vi "YAML to Elements.vi"(8 "error in (no error)":errorcluster, 10 "Parser State":T4) -> (0 "error out":errorcluster, 2 "Elements":T1[](array[typedef]))   [LabVIEW 2020, in "CDM-Config.lvlib" / "Config-YAML.lvclass"]
uses:
  Config-YAML.lvclass
  Config-YAML.lvclass/Config-YAML.ctl
  Value Type.ctl
  CDM-Config.lvlib
  Parser State.ctl
  Meta Data.ctl
  Config Element.ctl
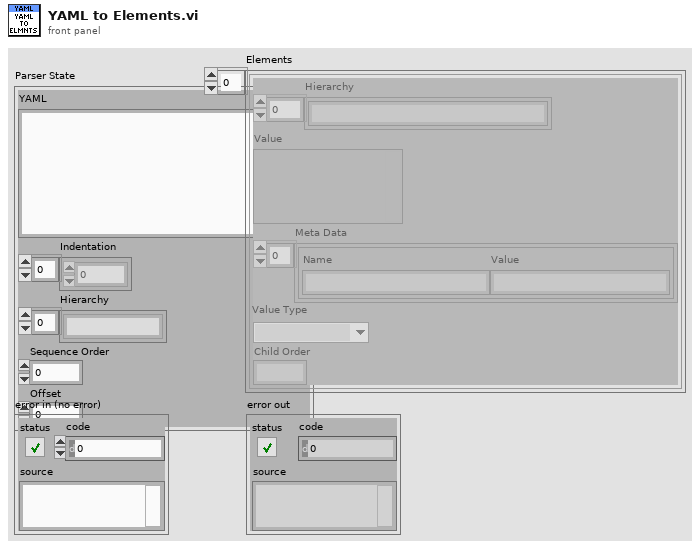
[diagram p1: front panel]
types:
  T1 = typedef "CDM-Config.lvlib/Config Element.ctl" = cluster{"Hierarchy":string[], "Value":variant, "Meta Data":T2[], "Value Type":T3, "Child Order":i32}
  T2 = typedef "CDM-Config.lvlib/Meta Data.ctl" = cluster{"Name":string, "Value":string}
  T3 = typedef "CDM-Config.lvlib/Value Type.ctl" = enum16{"String", "Number", "Bool", "Object", "Array"}
  T4 = typedef "CDM-Config.lvlib/Config-YAML.lvclass/Parser State.ctl" = cluster{"YAML":string, "Indentation":i32[], "Hierarchy":string[], "Sequence Order":i32, "Offset":i32}
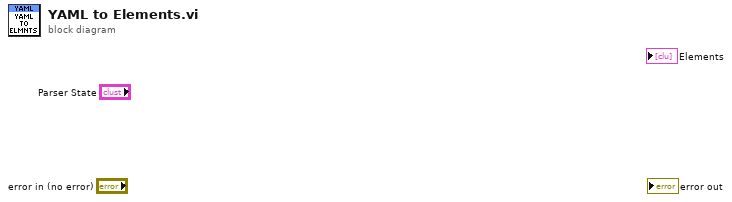
[diagram p0: block diagram]
diagram:
